vi "FTW-Collection-JSON-Serialize.vi"(0 "Collection":refnum<class "FTW-Collection.lvclass">, 5 "Whitespace Delimiter (after commas)":string="\n ", 11 "error in":errorcluster) -> (4 "Collection out":refnum<class "FTW-Collection.lvclass">, 6 "Serialized Collection":string, 15 "error out":errorcluster)   [LabVIEW 2012, in "FTW-Collection.lvclass"]
uses:
  FTW-Collection.lvclass
panel:
  # "Inputs"
  # "Outputs"
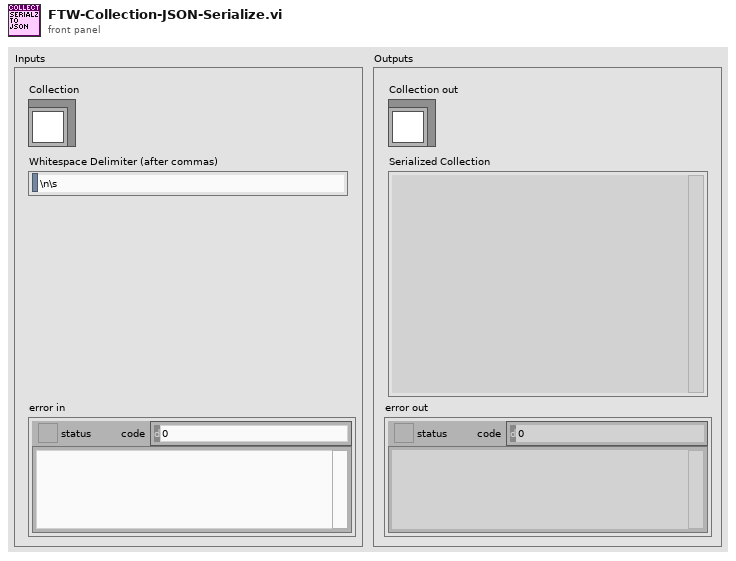
[diagram p1: front panel]
types:
  T1 = typedef "FTW-Collection-KeyValuePair.ctl" = cluster{"Key":string, "Value":string}
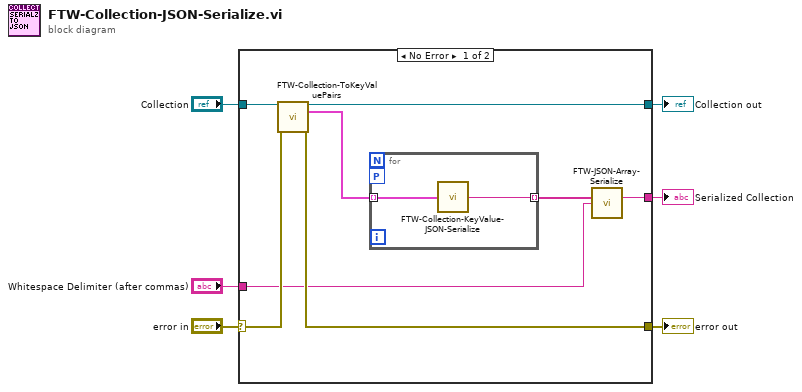
[diagram p0: block diagram]
diagram:
  n1 = case shown="No Error" "error in" {
    selector: "error in" -> [w12 w18]
    tunnel: [w11 w18] -> w6
    tunnel: "Collection" -> [w14 w17]
    tunnel: [w13 w17] -> w3
    tunnel: [w8 _] -> w2
    tunnel: "Whitespace Delimiter (after commas)" -> [w7 _]
    frame No Error {
      n2 = call "FTW-Collection-ToKeyValuePairs.vi"("Collection"=w14, "error in"=w12) -> ("Collection out"=w13:refnum<class "FTW-Collection.lvclass">, "Key-Value Pairs"=w10:T1[], "error out"=w11:errorcluster)  [unwired: 11 in]
      n3 = for {
        tunnel: [w15] -> w9 mode=indexing
        tunnel: w10 -> [w16] mode=indexing
        workers-P: _ -> [_]
        n4 = call "FTW-Collection-KeyValue-JSON-Serialize.vi"("Key-Value Pair"=w16) -> ("Serialized Key-Value Pair"=w15:string)
      }
      n5 = call "FTW-JSON-Array-Serialize.vi"("Array of JSON Elements"=w9, "Whitespace Delimiter (after commas)"=w7) -> ("JSON Array"=w8:string)  [unwired: 13 in]
    }
    frame Error {
    }
  }
  "error out" <- w6
  "Serialized Collection" <- w2
  "Collection out" <- w3
